vi "DAQ_Initialization.vi"(8 "error in (no error)":errorcluster) -> (0 "error out":errorcluster={"status"=TRUE, "code"=-200220, "source"="DAQmx Create Channel (CO-Pulse Generation-Time).vi:7440001<append>\n<B>Device Specified: </B>USB-6363\n<B>Suggested Device(s): </B>USB-6353\n\n<B>Task Name: </B>_unnamedTask<2>"})   [LabVIEW 2025]
uses:
  <vilib>/DAQmx/create/channels.llb/DAQmx Create Channel (CO-Pulse Generation-Time).vi
  <vilib>/DAQmx/create/channels.llb/DAQmx Create Channel (DO-Digital Output).vi
  <vilib>/DAQmx/configure/timing.llb/DAQmx Timing (Sample Clock).vi
  <vilib>/DAQmx/configure/trigger.llb/DAQmx Start Trigger (Digital Edge).vi
  <vilib>/DAQmx/create/channels.llb/DAQmx Create Channel (AO-Voltage-Basic).vi
  <resource>/objmgr/daqmx.rc
panel:
  in  "AO | Z":tag="USB-6353/ao3"
  in  "AO | Pockels":tag="USB-6353/ao2"
  in  "AO | Lasers":tag="USB-6353/ao0:1"
  in  "Trigger":tag="/USB-6353/PFI12"
  in  "DO":tag="USB-6353/port0/line0:3"
  in  "Counter":tag="USB-6353/ctr0"
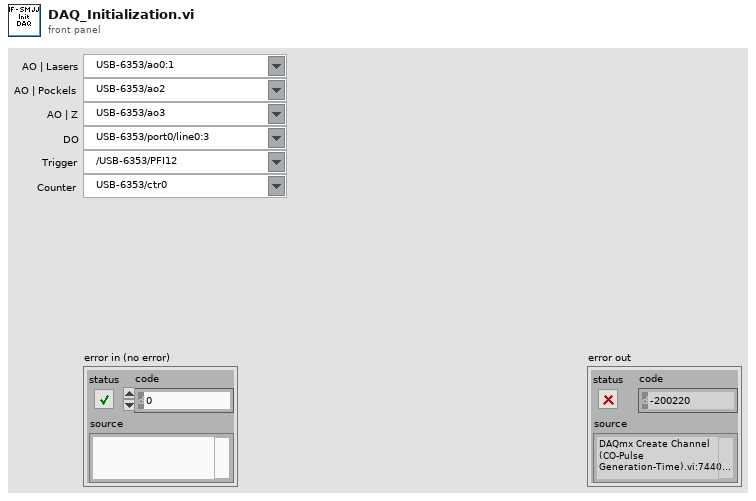
[diagram p1: front panel]
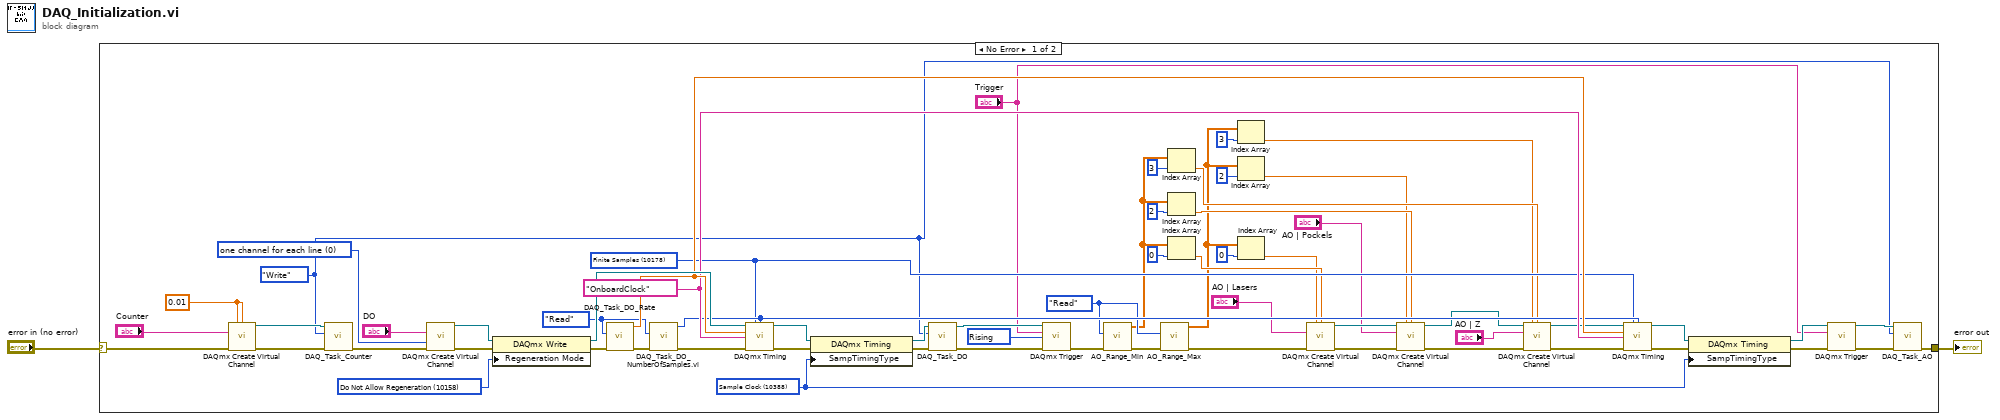
[diagram p0: block diagram]
diagram:
  n1 = case shown="No Error" "error in (no error)" {
    selector: "error in (no error)" -> [w45 w67]
    tunnel: [w33 w67] -> w2
    frame No Error {
      w20 = enum16{"Init", "Write", "Read"}."Read" ("Action")
      w23 = enum16{"Init", "Write", "Read"}."Read" ("Action")
      w24 = enum16{"Init", "Write", "Read"}."Write" ("Action")
      w42 = tag "OnboardClock" ("Timing source")
      w66 = 0 items=["one channel for each line", "one channel for all lines"] ("line grouping")
      w39 = 10388 items=["Sample Clock"=10388, "Burst Handshake"=12548, "Handshake"=10389, "Implicit"=10451, "On Demand"=10390, "Change Detection"=12504, "Pipelined Sample Clock"=14668] ("SampTimingType")
      w40 = 10178 items=["Finite Samples"=10178, "Continuous Samples"=10123] ("sample mode")
      w56 = 10158 items=["Allow Regeneration"=10097, "Do Not Allow Regeneration"=10158] ("RegenMode")
      w54 = 10280 items=["Rising"=10280, "Falling"=10171] ("edge")
      w53 = 0.01 ("low time")
      n2 = call-poly <vilib>:"DAQmx Create Virtual Channel.vi"("high time"=w53, "low time"=w53, "counter"="Counter", "error in"=w45) -> ("task out"=w49:refnum<k21>, "error out"=w48:errorcluster)  [unwired: 10 in]
      n3 = call "DAQ_Task_Counter.vi"("error in"=w48, "Action"=w24, "DAQ_Task_Counter"=w49) -> ("error out"=w50:errorcluster)  [unwired: 7 in, 1 out]
      n4 = call-poly <vilib>:"DAQmx Create Virtual Channel.vi"("lines"="DO", "line grouping"=w66, "error in"=w50) -> ("task out"=w58:refnum<k21>, "error out"=w57:errorcluster)  [unwired: 11 in]
      n5 = property class="DAQmx Write"(reference=w58, error in=w57, "Regeneration Mode"=w56) -> (reference out=w55:refnum<k21>, error out=w63:errorcluster)
      n6 = call "DAQ_Task_DO_Rate.vi"("error in"=w63, "Action"=w23) -> ("error out"=w64:errorcluster, "DO_Rate"=w43:dbl)  [unwired: 8 in]
      n7 = call "DAQ_Task_DO_NumberOfSamples.vi.vi"("error in"=w64, "Action"=w23) -> ("error out"=w65:errorcluster, "Samples"=w41:u32)  [unwired: 8 in]
      n8 = call-poly <vilib>:"DAQmx Timing.vi"("task/channels in"=w55, "sample mode"=w40, "samples per channel"=w41, "rate"=w43, "source"=w42, "error in"=w65) -> ("task out"=w61:refnum<k21>, "error out"=w60:errorcluster)  [unwired: 8 in]
      n9 = property class="DAQmx Timing"(reference=w61, error in=w60, "SampTimingType"=w39) -> (reference out=w62:refnum<k21>, error out=w59:errorcluster)
      n10 = call "DAQ_Task_DO.vi"("error in"=w59, "Action"=w24, "DAQ_Task_DO"=w62) -> ("error out"=w52:errorcluster, "DAQ_Task_DO"=w51:refnum<k21>)  [unwired: 7 in]
      n11 = call-poly <vilib>:"DAQmx Trigger.vi"("task/channels in"=w51, "source"="Trigger", "edge"=w54, "error in"=w52) -> ("error out"=w3:errorcluster)  [unwired: 10 in, 1 out]
      n12 = call "AO_Range_Min.vi"("error in"=w3, "Action"=w20) -> ("error out"=w22:errorcluster, "AO | Min"=w19:dbl[])  [unwired: 8 in]
      n13 = call "AO_Range_Max.vi"("error in"=w22, "Action"=w20) -> ("error out"=w21:errorcluster, "AO | Max"=w9:dbl[])  [unwired: 8 in]
      n14 = Index Array(array=w19, index=3) -> (element=w13:dbl)
      n15 = Index Array(array=w19, index=2) -> (element=w14:dbl)
      n16 = Index Array(array=w19, index=0) -> (element=w15:dbl)
      n17 = Index Array(array=w9, index=3) -> (element=w6:dbl)
      n18 = Index Array(array=w9, index=2) -> (element=w7:dbl)
      n19 = Index Array(array=w9, index=0) -> (element=w8:dbl)
      n20 = call-poly <vilib>:"DAQmx Create Virtual Channel.vi"("maximum value"=w8, "minimum value"=w15, "physical channels"="AO | Lasers", "error in"=w21) -> ("task out"=w44:refnum<k21>, "error out"=w5:errorcluster)  [unwired: 10 in]
      n21 = call-poly <vilib>:"DAQmx Create Virtual Channel.vi"("task in"=w44, "maximum value"=w7, "minimum value"=w14, "physical channels"="AO | Pockels", "error in"=w5) -> ("task out"=w28:refnum<k21>, "error out"=w4:errorcluster)  [unwired: 9 in]
      n22 = call-poly <vilib>:"DAQmx Create Virtual Channel.vi"("task in"=w28, "maximum value"=w6, "minimum value"=w13, "physical channels"="AO | Z", "error in"=w4) -> ("task out"=w27:refnum<k21>, "error out"=w26:errorcluster)  [unwired: 9 in]
      n23 = call-poly <vilib>:"DAQmx Timing.vi"("task/channels in"=w27, "sample mode"=w40, "samples per channel"=w41, "rate"=w43, "source"=w42, "error in"=w26) -> ("task out"=w31:refnum<k21>, "error out"=w32:errorcluster)  [unwired: 8 in]
      n24 = property class="DAQmx Timing"(reference=w31, error in=w32, "SampTimingType"=w39) -> (reference out=w38:refnum<k21>, error out=w37:errorcluster)
      n25 = call-poly <vilib>:"DAQmx Trigger.vi"("task/channels in"=w38, "source"="Trigger", "error in"=w37) -> ("task out"=w35:refnum<k21>, "error out"=w34:errorcluster)  [unwired: 11 in]
      n26 = call "DAQ_Task_AO.vi"("error in"=w34, "Action"=w24, "DAQ_Task_DO"=w35) -> ("error out"=w33:errorcluster)  [unwired: 7 in, 1 out]
    }
    frame Error {
    }
  }
  "error out" <- w2
